vi "选择表格的行并改变背景颜色.vi"() -> ()   [LabVIEW 2012]
uses:
  <vilib>/Utility/miscctls.llb/LVRowAndColumnTypeDef.ctl
panel:
  out "选中的行":string[](array[string])
  in  "表格控件":string[][](table)
  in  "停止":bool
  out "单元格位置":T1
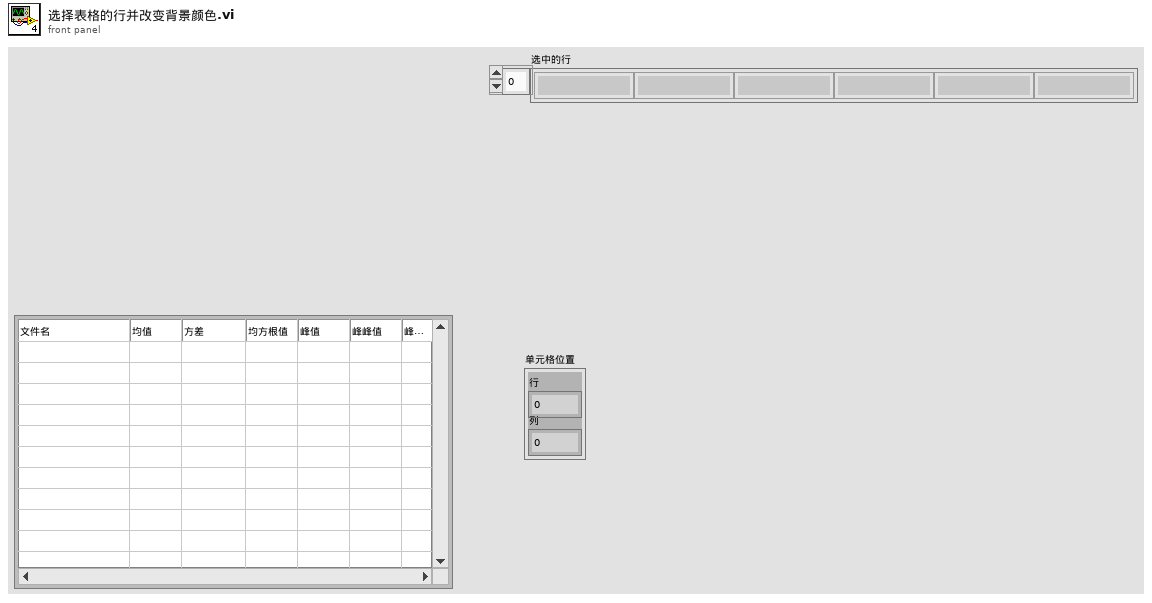
[diagram p1: front panel]
types:
  T1 = typedef "LVRowAndColumnTypeDef.ctl" = cluster{"Row":i32, "Column":i32}
  T2 = typedef "LVPoint32TypeDef.ctl" = cluster{"Horizontal":i32, "Vertical":i32}
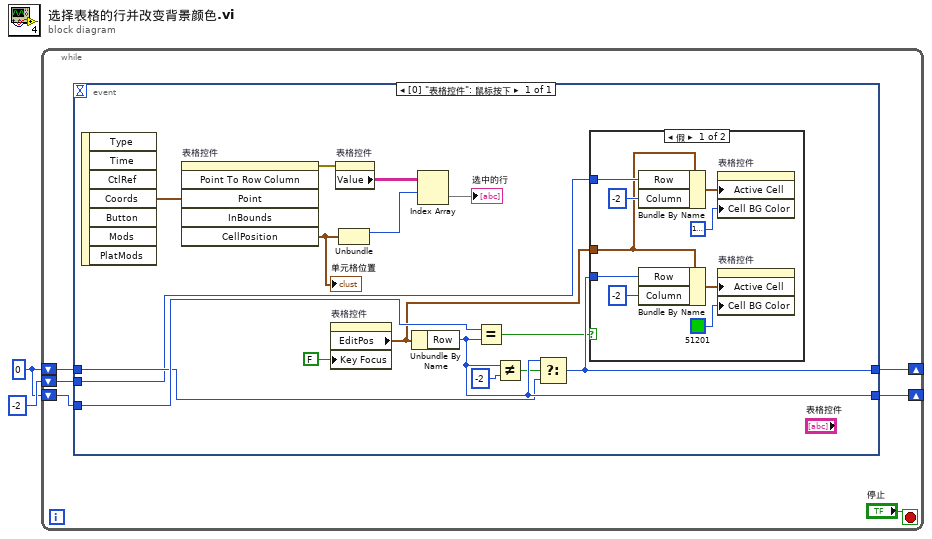
[diagram p0: block diagram]
diagram:
  w1 = 0 ("Row")
  n1 = while {
    shift-right: [w7] -> _
    shift-left: w1 -> [w5]
    shift-right: [w6] -> _
    shift-left: w1 -> [w4]
    shift-left: -2 ("Row") -> [w3]
    stop <- "停止" stop-if-true
    n2 = event shown="[0] \"表格控件\": 鼠标按下" {
      selector: _ -> [_]
      dyn-events: _ -> [_]
      timeout: _ -> [_]
      tunnel: [w18] -> w7
      tunnel: [w17] -> w6
      tunnel: w5 -> [w16]
      tunnel: w4 -> [w15]
      tunnel: w3 -> [w14]
      event "表格控件": Mouse Down {
        n3 = event-data() -> ("Coords"=w23:T2)  [unwired: 1 in, 6 out]
        n4 = invoke on="表格控件" class="Tbl (严格)" method="Point To Row Column"("Point"=w23) -> (error out=w22:errorcluster, "CellPosition"=w19:T1)  [unwired: 5 in, 4 out]
        "单元格位置" <- w19
        n5 = property on="表格控件" class="Tbl (严格)"("Key Focus"=FALSE ("键选中")) -> ("EditPos"=w10:T1)  [unwired: 2 in, 2 out]
        n6 = property on="表格控件" class="Tbl (严格)"(error in=w22) -> ("Value"=w21:string[][])  [unwired: 1 in, 2 out]
        n7 = Unbundle(w19) -> ("Row"=w24:i32)  [unwired: 1 out]
        n8 = Unbundle By Name(w10) -> ("Row"=w18:i32)
        n9 = Index Array(array=w21, index (row)=w24) -> (element=→"选中的行":string[])  [unwired: 1 in]
        n10 = Equal?(x=w16, y=w18) -> (x = y?=w11:bool)
        n11 = Not Equal?(x=w18, y=-2 ("Column")) -> (x != y?=w12:bool)
        n12 = Select(t=w18, s=w12, f=w15) -> (s? t:f=w17:i32)
        n13 = case shown="假" w11 {
          tunnel: w17 -> [w32 _]
          tunnel: w14 -> [w30 _]
          tunnel: w10 -> [w29 _]
          frame False {
            n14 = Bundle By Name(cluster=w29, "Row"=w30, "Column"=-2) -> (w28:T1)
            n15 = Bundle By Name(cluster=w29, "Row"=w32, "Column"=-2) -> (w26:T1)
            n16 = property on="表格控件" class="Tbl (严格)"("Active Cell"=w28, "Cell BG Color"=u32 16777226) -> ()  [unwired: 2 in, 2 out]
            n17 = property on="表格控件" class="Tbl (严格)"("Active Cell"=w26, "Cell BG Color"=u32 51201) -> ()  [unwired: 2 in, 2 out]
          }
          frame True {
          }
        }
      }
    }
  }
